vi "Is a Dqmh Module.vi"(8 "error in":errorcluster, 11 "Library Ref":refnum<vi>) -> (0 "error out":errorcluster, 2 "Is Cloneable":bool, 3 "Is Dqmh Module":bool)   [LabVIEW 2021, in "TAF Proj Document Type.lvlib" / "Project Parser.lvlib"]
uses:
  <vilib>/Wovalab/AntiDoc/Document Type/Add-ons/LabVIEW TAF Project/Project Parser/Project Parser.lvlib
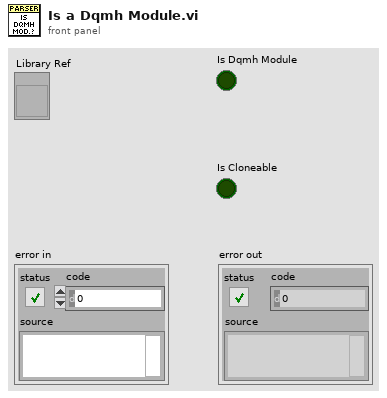
[diagram p1: front panel]
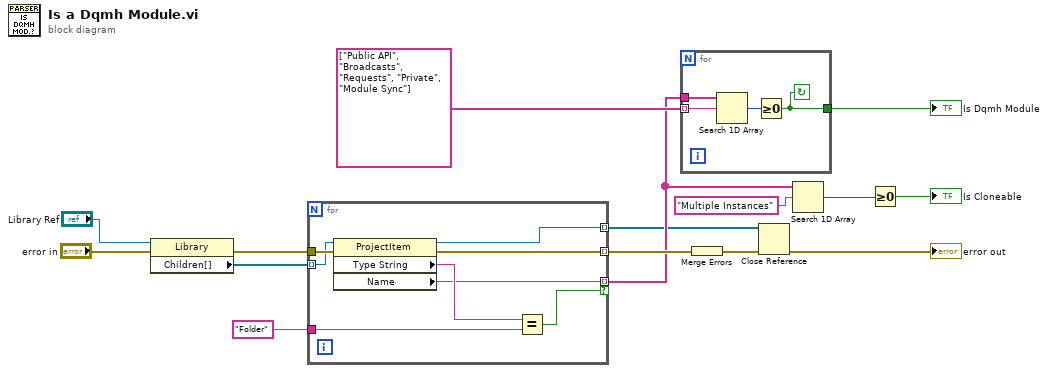
[diagram p0: block diagram]
diagram:
  n1 = property class="Library"(reference="Library Ref", error in="error in") -> (error out=w1:errorcluster, "Children[]"=w4:refnum<vi>[])  [unwired: 1 out]
  n2 = for {
    tunnel: [w16] -> w11 mode=indexing if=w17
    tunnel: w1 -> [w23]
    tunnel: [w19] -> w14 mode=indexing
    tunnel: [w20] -> w6 mode=indexing
    tunnel: w4 -> [w22] mode=indexing
    tunnel: "Folder" ("Type") -> [w18]
    n3 = property class="ProjectItem"(reference=w22, error in=w23) -> (reference out=w20:refnum<vi>, error out=w19:errorcluster, "Type String"=w21:string, "Name"=w16:string)
    n4 = Equal?(x=w21, y=w18) -> (x = y?=w17:bool)
  }
  n5 = for {
    tunnel: string[] ["Public API", "Broadcasts", "Requests", "Private", "Module Sync"] -> [w27] mode=indexing
    tunnel: w11 -> [w26]
    tunnel: [w24] -> w12
    stop <- w24 continue-if-true
    n6 = Search 1D Array(1D array=w26, element=w27) -> (index of element=w25:i32)  [unwired: 1 in]
    n7 = Greater Or Equal To 0?(x=w25) -> (x >= 0?=w24:bool)
  }
  "Is Dqmh Module" <- w12
  n8 = Merge Errors(w14) -> (w15:errorcluster)
  n9 = Close Reference(reference=w6, error in (no error)=w15) -> (error out=→"error out":errorcluster)
  n10 = Search 1D Array(1D array=w11, element="Multiple Instances") -> (index of element=w9:i32)  [unwired: 1 in]
  n11 = Greater Or Equal To 0?(x=w9) -> (x >= 0?=→"Is Cloneable":bool)
